vi "Drive_Utils_DistanceRadiusToLeftRight.vi"(4 "Turn Radius":dbl, 5 "Distance":dbl) -> (1 "Right Distance":dbl, 2 "Left Distance":dbl)   [LabVIEW 2009, in "Drive.lvlib" / "Drive_Utils.lvlib"]
uses:
  Drive_Utils.lvlib
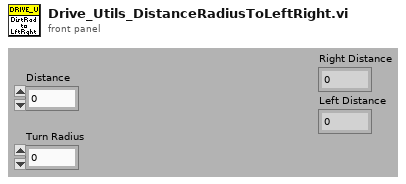
[diagram p1: front panel]
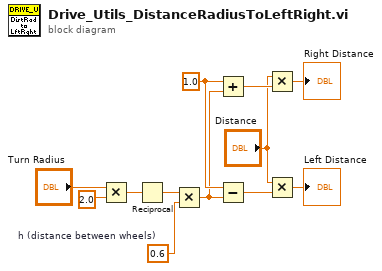
[diagram p0: block diagram]
diagram:
  w5 = 1.0 ("y")
  w8 = 0.6  # h (distance between wheels)
  n1 = Multiply(x="Turn Radius", y=2.0) -> (x*y=w10:dbl)
  n2 = Reciprocal(x=w10) -> (1/x=w9:dbl)
  n3 = Multiply(x=w9, y=w8) -> (x*y=w4:dbl)
  n4 = Add(x=w5, y=w4) -> (x+y=w7:dbl)
  n5 = Subtract(x=w5, y=w4) -> (x-y=w2:dbl)
  n6 = Multiply(x="Distance", y=w7) -> (x*y=→"Right Distance":dbl)
  n7 = Multiply(x="Distance", y=w2) -> (x*y=→"Left Distance":dbl)
